vi "Copy Speed Test.vi"() -> ()   [LabVIEW 2019, in "LV-Data.PGSQL.lvclass"]
uses:
  LV-Data.PGSQL.lvclass
panel:
  in  "table":string="twenty_doubes"
  in  "Path to data csv":path=path "C:/Users/Phil/Desktop/jack/data_speed_test.csv"
  out "Time (s)":dbl
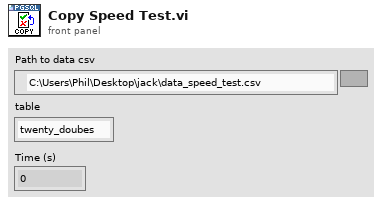
[diagram p1: front panel]
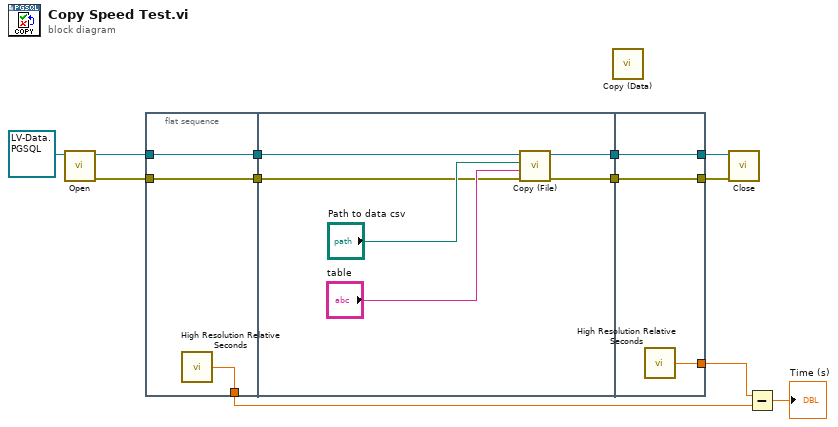
[diagram p0: block diagram]
diagram:
  n1 = call-dynamic "Open.vi"("Data.PG in"=refnum<class "LV-Data.PGSQL.lvclass"> refnum) -> ("error out"=w8:errorcluster, "Data.PG out"=w6:refnum<class "LV-Data.PGSQL.lvclass">)  [unwired: 9 in]
  n2 = flat-sequence {
    tunnel: [w15] -> w11
    tunnel: [w14] -> w9
    tunnel: w8 -> [w14]
    tunnel: [w13] -> w7
    tunnel: w6 -> [w13]
    tunnel: w9 -> [w19]
    tunnel: w7 -> [w18]
    tunnel: [w17] -> w4
    tunnel: [w16] -> w2
    tunnel: [w24] -> w12
    tunnel: [w23] -> w5
    tunnel: w4 -> [w23]
    tunnel: [w22] -> w3
    tunnel: w2 -> [w22]
    frame #0 {
      n3 = call <vilib>:"High Resolution Relative Seconds.vi"() -> ("relative seconds"=w15:dbl)
    }
    frame #1 {
      n4 = call "Copy (File).vi"("error in (no error)"=w19, "table"="table", "Path to spreadsheet"="Path to data csv", "Data.PGSQL"=w18) -> ("error out"=w17:errorcluster, "Data.PGSQL out"=w16:refnum<class "LV-Data.PGSQL.lvclass">)  [unwired: 6 in]
    }
    frame #2 {
      n5 = call <vilib>:"High Resolution Relative Seconds.vi"() -> ("relative seconds"=w24:dbl)
    }
  }
  n6 = call "Copy (Data).vi"() -> ()  [unwired: 10 in, 2 out]
  n7 = call-dynamic "Close.vi"("error in (no error)"=w5, "Data.PG in"=w3) -> ()  [unwired: 8 in, 2 out]
  n8 = Subtract(x=w12, y=w11) -> (x-y=→"Time (s)":dbl)
